vi "Revision Query.vi"(8 "error in (no error)":errorcluster, 11 "VISA resource name":refnum<visa-resource-name>) -> (0 "error out":errorcluster, 1 "Instrument Firmware Revision":string, 2 "Instrument Driver Revision":string, 3 "VISA resource name out":refnum<visa-resource-name>)   [LabVIEW 2012, in "MicroStrain 3DM-GXx.lvlib"]
doc: "Queries the current instrument firmware revision and instrument driver revision.\n\nRefer to the Readme file for detailed driver information including modification history."
uses:
  <instrlib>/MicroStrain 3DM-GXx/MicroStrain 3DM-GXx.lvlib
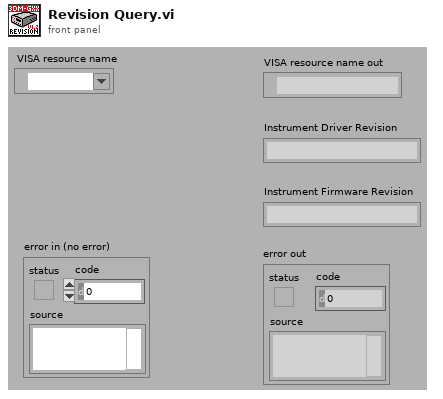
[diagram p1: front panel]
types:
  T1 = enum32{"invalid app kind", "Development System", "Run Time System", "Student Edition", "Embedded LabVIEW", "Evaluation", "Custom"}
  T2 = cluster{"Major":u16, "Minor":u16, "Fix":u16, "Build":u16}
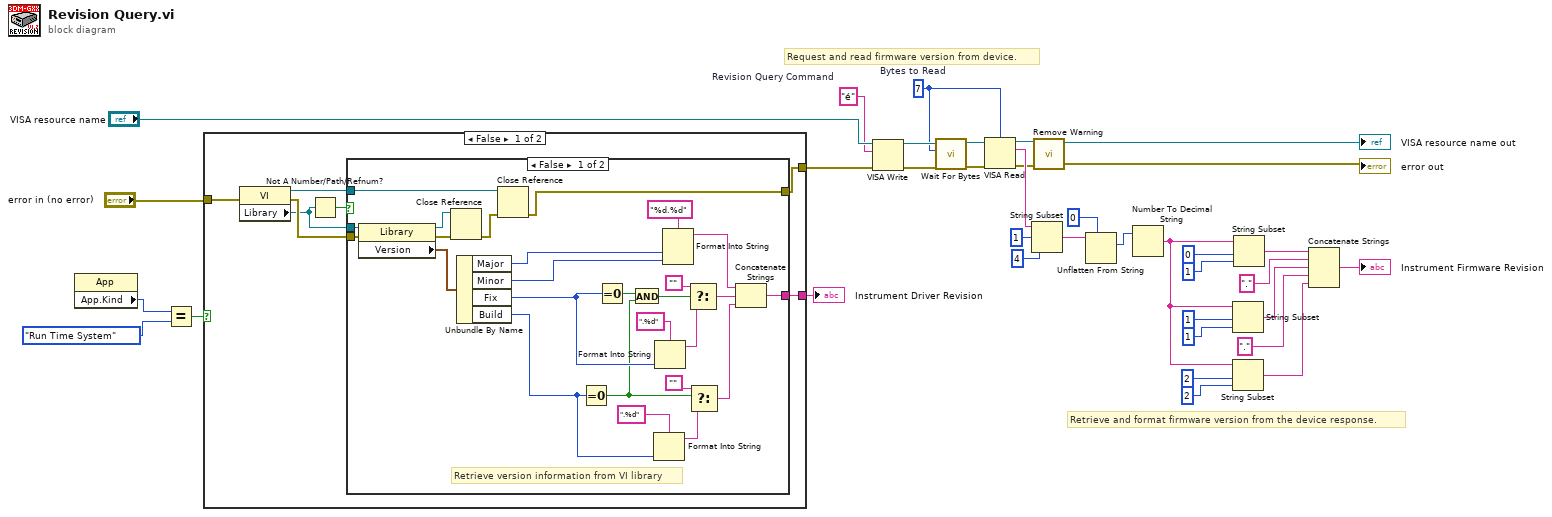
[diagram p0: block diagram]
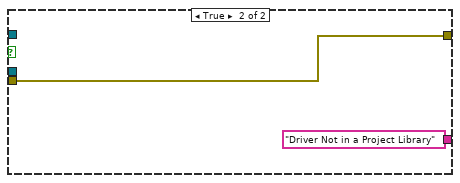
[diagram p2: hidden frame]
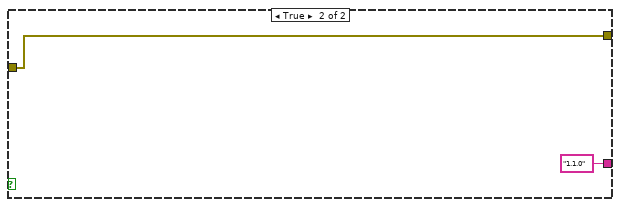
[diagram p3: hidden frame]
diagram:
  w35 = "é"  # Revision Query Command
  w24 = u32 7  # Bytes to Read
  # "Retrieve and format firmware version from the device response."
  # "Request and read firmware version from device."
  n1 = property class="App"() -> ("App.Kind"=w30:T1)  [unwired: 2 in, 2 out]
  n2 = Equal?(x=w30, y=T1."Run Time System" ("Application:Kind")) -> (x = y?=w31:bool)
  n3 = case shown="False" w31 {
    tunnel: [w39 "1.1.0"] -> w34
    tunnel: "error in (no error)" -> [w38 w72]
    tunnel: [w37 w72] -> w32
    frame False {
      n4 = property class="VI"(error in=w38) -> (reference out=w43:refnum<vi>, error out=w42:errorcluster, "Library"=w41:refnum<vi>)  [unwired: 1 in]
      n5 = Not A Number/Path/Refnum?(number/path/refnum=w41) -> (NaN/Path/Refnum?=w40:bool)
      n6 = case shown="False" w40 {
        tunnel: w43 -> [w66 _]
        tunnel: w42 -> [w51 w71]
        tunnel: [w46 w71] -> w37
        tunnel: [w45 "Driver Not in a Project Library"] -> w39
        tunnel: w41 -> [w44 _]
        frame False {
          # "Retrieve version information from VI library"
          n7 = property class="Library"(reference=w44, error in=w51) -> (reference out=w68:refnum<vi>, error out=w69:errorcluster, "Version"=w65:T2)
          n8 = Close Reference(reference=w68, error in (no error)=w69) -> (error out=w67:errorcluster)
          n9 = Unbundle By Name(w65) -> ("Major"=w54:u16, "Minor"=w53:u16, "Fix"=w50:u16, "Build"=w52:u16)
          n10 = Close Reference(reference=w66, error in (no error)=w67) -> (error out=w46:errorcluster)
          n11 = Equal To 0?(x=w52) -> (x = 0?=w48:bool)
          n12 = Equal To 0?(x=w50) -> (x = 0?=w49:bool)
          n13 = And(x=w49, y=w48) -> (x .and. y?=w47:bool)
          n14 = Format Into String(format string=".%d", w52) -> (resulting string=w58:string)  [unwired: 2 in, 1 out]
          n15 = Format Into String(format string=".%d", w50) -> (resulting string=w62:string)  [unwired: 2 in, 1 out]
          n16 = Format Into String(format string="%d.%d", w54, w53) -> (resulting string=w60:string)  [unwired: 2 in, 1 out]
          n17 = Select(t="", s=w47, f=w62) -> (s? t:f=w59:string)
          n18 = Select(t="", s=w48, f=w58) -> (s? t:f=w55:string)
          n19 = Concatenate Strings(w60, w59, w55) -> (w45:string)
        }
        frame True {
        }
      }
    }
    frame True {
    }
  }
  "Instrument Driver Revision" <- w34
  n20 = VISA Write(VISA resource name="VISA resource name", write buffer=w35, error in (no error)=w32) -> (VISA resource name out=w28:refnum<visa-resource-name>, error out=w25:errorcluster)  [unwired: 1 out]
  n21 = call <instrlib>:"Wait For Bytes.vi"("error in (no error)"=w25, "Bytes To Read (0)"=w24, "VISA resource name"=w28) -> ("error out"=w26:errorcluster, "VISA resource name out"=w27:refnum<visa-resource-name>)  [unwired: 7 in]
  n22 = VISA Read(VISA resource name=w27, byte count=w24, error in (no error)=w26) -> (VISA resource name out=w4:refnum<visa-resource-name>, read buffer=w20:string, error out=w1:errorcluster)  [unwired: 1 out]
  n23 = String Subset(string=w20, offset (0)=1, length (rest)=4 ("length (rest)")) -> (substring=w18:string)
  n24 = call <instrlib>:"Remove Warning.vi"("error in (no error)"=w1, "VISA resource name"=w4) -> ("error out"=→"error out":errorcluster, "VISA resource name out"=→"VISA resource name out":refnum<visa-resource-name>)  [unwired: 2 in]
  n25 = Unflatten From String(type=u32 0, binary string=w18) -> (value=w19:u32)  [unwired: 3 in, 2 out]
  n26 = Number To Decimal String(number=w19) -> (decimal integer string=w11:string)  [unwired: 1 in]
  n27 = String Subset(string=w11, offset (0)=1, length (rest)=1 ("length (rest)")) -> (substring=w10:string)
  n28 = String Subset(string=w11, offset (0)=2, length (rest)=2 ("length (rest)")) -> (substring=w8:string)
  n29 = String Subset(string=w11, offset (0)=0, length (rest)=1 ("length (rest)")) -> (substring=w15:string)
  n30 = Concatenate Strings(w15, "." ("string"), w10, "." ("string"), w8) -> (→"Instrument Firmware Revision":string)
